vi "WorkingCode2.vi"() -> ()   [LabVIEW 2013]
panel:
  out "Com Id 2":i32=-1
  out "Connected \nRobotino 2":bool
  in  "Disconnect":bool
  in  "Omega":sgl
  out "Motor 3 Speed":sgl
  out "Motor 2 Speed":sgl
  out "Motor 1 Speed":sgl
  in  "Velocity X":sgl
  out "error out":errorcluster
  out "Input 4":bool
  out "Input 3":bool
  out "Input 2":bool
  out "Input 1":bool
  out "Com Id 1":i32=-1
  in  "Robotino IP":string="127.0.0.1:8080"
  out "Connected\nRobotino":bool
  in  "Connect":bool
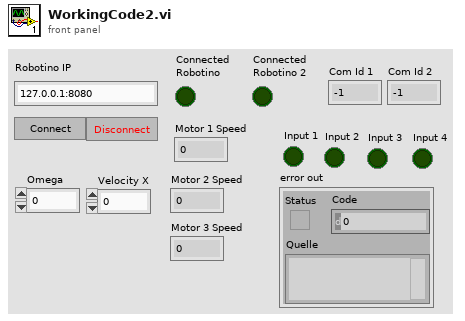
[diagram p1: front panel]
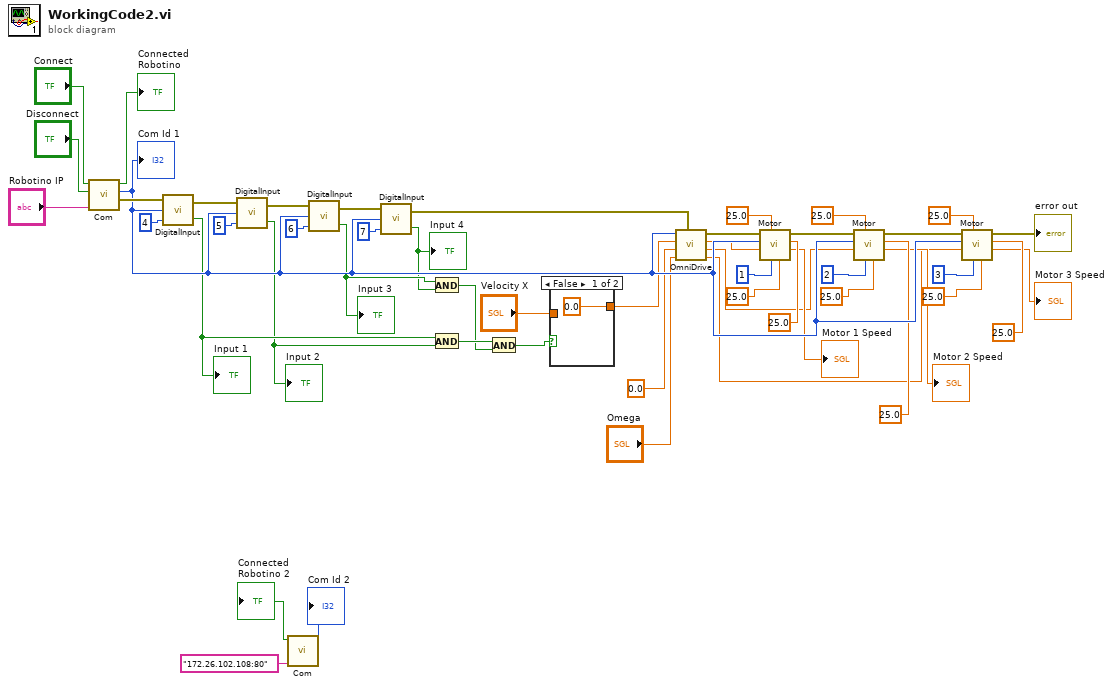
[diagram p0: block diagram]
diagram:
  n1 = call <userlib>:"Com.vi"("Hostname"="Robotino IP", "Disconnect"="Disconnect", "Connect"="Connect") -> ("error out"=w47:errorcluster, "Com Id"=w35:i32, "Connected"=→"Connected\nRobotino":bool)  [unwired: 1 in, 1 out]
  "Com Id 1" <- w35
  n2 = call <userlib>:"DigitalInput.vi"("Digital \nInput Number"=u32 4 ("Digital \nInput Number"), "Com Id"=w35, "error in (no error)"=w47) -> ("Input"=w10:bool, "error out"=w46:errorcluster)
  "Input 1" <- w10
  n3 = call <userlib>:"DigitalInput.vi"("Digital \nInput Number"=u32 5 ("Digital \nInput Number"), "Com Id"=w35, "error in (no error)"=w46) -> ("Input"=w9:bool, "error out"=w45:errorcluster)
  "Input 2" <- w9
  n4 = call <userlib>:"Com.vi"("Hostname"="172.26.102.108:80") -> ("Com Id"=→"Com Id 2":i32, "Connected"=→"Connected \nRobotino 2":bool)  [unwired: 3 in, 2 out]
  n5 = call <userlib>:"DigitalInput.vi"("Digital \nInput Number"=u32 6 ("Digital \nInput Number"), "Com Id"=w35, "error in (no error)"=w45) -> ("Input"=w5:bool, "error out"=w44:errorcluster)
  "Input 3" <- w5
  n6 = call <userlib>:"DigitalInput.vi"("Digital \nInput Number"=u32 7 ("Digital \nInput Number"), "Com Id"=w35, "error in (no error)"=w44) -> ("Input"=w4:bool, "error out"=w39:errorcluster)
  "Input 4" <- w4
  n7 = And(x=w5, y=w4) -> (x .and. y?=w6:bool)
  n8 = And(x=w10, y=w9) -> (x .and. y?=w8:bool)
  n9 = And(x=w8, y=w6) -> (x .and. y?=w7:bool)
  n10 = case shown="False" w7 {
    tunnel: "Velocity X" -> [_ w52]
    tunnel: [sgl 0.0 ("Velocity X") w52] -> w12
    frame False {
    }
    frame True {
    }
  }
  n11 = call <userlib>:"OmniDrive.vi"("error in (no error)"=w39, "Omega"="Omega", "Velocity Y"=sgl 0.0, "Velocity X"=w12, "Com Id"=w35) -> ("Motor Speed 3"=w14:sgl, "Motor Speed 2"=w15:sgl, "Motor Speed 1"=w16:sgl, "error out"=w38:errorcluster)  [unwired: 1 in]
  n12 = call <userlib>:"Motor.vi"("kd"=sgl 25.0, "ki"=sgl 25.0, "Motor Number"=1, "kp"=sgl 25.0, "Speed"=w16, "Com Id"=w35, "error in (no error)"=w38) -> ("Actual Speed"=→"Motor 1 Speed":sgl, "error out"=w37:errorcluster)  [unwired: 1 in, 2 out]
  n13 = call <userlib>:"Motor.vi"("kd"=sgl 25.0, "ki"=sgl 25.0, "Motor Number"=2, "kp"=sgl 25.0, "Speed"=w15, "Com Id"=w35, "error in (no error)"=w37) -> ("Actual Speed"=→"Motor 2 Speed":sgl, "error out"=w36:errorcluster)  [unwired: 1 in, 2 out]
  n14 = call <userlib>:"Motor.vi"("kd"=sgl 25.0, "ki"=sgl 25.0, "Motor Number"=3, "kp"=sgl 25.0, "Speed"=w14, "Com Id"=w35, "error in (no error)"=w36) -> ("Actual Speed"=→"Motor 3 Speed":sgl, "error out"=→"error out":errorcluster)  [unwired: 1 in, 2 out]
